vi "servo_control.vi"() -> ()   [LabVIEW 2018]
uses:
  <vilib>/LabVIEW Interface for Arduino/Type Defs/Board Type.ctl
  <vilib>/LabVIEW Interface for Arduino/Type Defs/Arduino Resource.ctl
  <vilib>/LabVIEW Interface for Arduino/Type Defs/Connection Type.ctl
  <vilib>/LabVIEW Interface for Arduino/LabVIEW Interface for Arduino.lvlib
panel:
  in  "stop":bool
  out "Angle moved 2":u8=15
  in  "Angle (Degrees) 2":u8(knob)=15 scale=0.0..180.0
  out "error out 2":errorcluster
  out "Arduino Resource":T1={"VISA resource"="", "Board Type"=enum."Uno", "Connection Type"=enum."USB / Serial", "Bytes Per Packet (15)"=15}
  in  "Baud Rate":u32=115200
  out "error out":errorcluster
  in  "Board Type (Uno)":T2
  out "Angle Moved":u8=15
  in  "Angle (Degrees)":u8(knob)=15 scale=0.0..180.0
  in  "VISA resource":refnum<visa-resource-name>
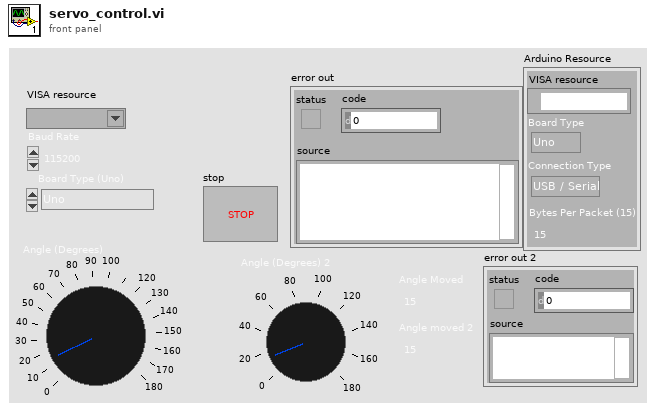
[diagram p1: front panel]
types:
  T1 = typedef "LabVIEW Interface for Arduino.lvlib/Arduino Resource.ctl" = cluster{"VISA resource":refnum<visa-resource-name>, "Board Type":T2, "Connection Type":enum8{"USB / Serial"}, "Bytes Per Packet (15)":u8}
  T2 = typedef "LabVIEW Interface for Arduino.lvlib/Board Type.ctl" = enum16{"Uno", "Dimuelanove w/Atmega 328", "Mega 2560"}
  T3 = typedef "LabVIEW Interface for Arduino.lvlib/Connection Type.ctl" = enum8{"USB / Serial", "XBEE", "BlueSmirf (Bluetooth)"}
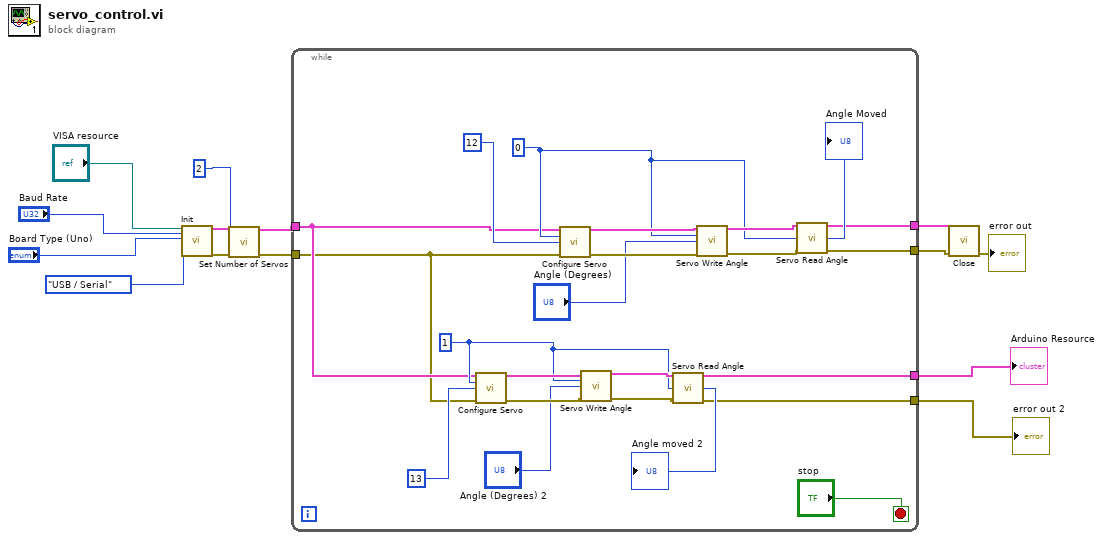
[diagram p0: block diagram]
diagram:
  n1 = call <vilib>:"Init.vi"("VISA resource"="VISA resource", "Baud Rate (115200)"="Baud Rate", "Board Type (Uno)"="Board Type (Uno)", "Connection Type (USB/Serial)"=Connection_Type."USB / Serial") -> ("Arduino Resource"=w9:T1, "error out"=w7:errorcluster)  [unwired: 14 in]
  n2 = call <vilib>:"Set Number of Servos.vi"("Arduino Resource"=w9, "Number Of Servos (1)"=u8 2, "error in"=w7) -> ("Arduino Resource"=w6:T1, "error out"=w5:errorcluster)  [unwired: 11 in]
  n3 = while {
    tunnel: w6 -> [w20]
    tunnel: w5 -> [w19]
    tunnel: [w18] -> w4
    tunnel: [w17] -> w3
    tunnel: [w16] -> w2
    tunnel: [w15] -> w1
    stop <- "stop" stop-if-true
    w25 = u8 1 ("Servo Number")
    w26 = u8 0 ("Servo Number (0)")
    n4 = call <vilib>:"Configure Servo.vi"("Arduino Resource"=w20, "Servo Number (0)"=w25, "DIO Pin (2)"=u8 13, "error in"=w19) -> ("Arduino Resource"=w30:T1, "error out"=w28:errorcluster)  [unwired: 10 in]
    n5 = call <vilib>:"Configure Servo.vi"("Arduino Resource"=w20, "Servo Number (0)"=w26, "DIO Pin (2)"=u8 12, "error in"=w19) -> ("Arduino Resource"=w36:T1, "error out"=w35:errorcluster)  [unwired: 10 in]
    n6 = call <vilib>:"Servo Write Angle.vi"("Arduino Resource"=w30, "Servo Number"=w25, "Angle (Degrees)"="Angle (Degrees) 2", "error in"=w28) -> ("Arduino Resource"=w29:T1, "error out"=w27:errorcluster)  [unwired: 10 in]
    n7 = call <vilib>:"Servo Read Angle.vi"("Arduino Resource"=w29, "Servo Number"=w25, "error in"=w27) -> ("Arduino Resource"=w15:T1, "Angle (Degrees)"=→"Angle moved 2":u8, "error out"=w16:errorcluster)  [unwired: 10 in]
    n8 = call <vilib>:"Servo Write Angle.vi"("Arduino Resource"=w36, "Servo Number"=w26, "Angle (Degrees)"="Angle (Degrees)", "error in"=w35) -> ("Arduino Resource"=w33:T1, "error out"=w32:errorcluster)  [unwired: 10 in]
    n9 = call <vilib>:"Servo Read Angle.vi"("Arduino Resource"=w33, "Servo Number"=w26, "error in"=w32) -> ("Arduino Resource"=w18:T1, "Angle (Degrees)"=→"Angle Moved":u8, "error out"=w17:errorcluster)  [unwired: 10 in]
  }
  "Arduino Resource" <- w1
  "error out 2" <- w2
  n10 = call <vilib>:"Close.vi"("Arduino Resource"=w4, "error in"=w3) -> ("error out"=→"error out":errorcluster)  [unwired: 13 in]
